vi "Broadcast Single Message.vi"(8 "error in (no error)":errorcluster, 10 "Message In":refnum<class "Message.lvclass">, 11 "Messenger in":refnum<class "Tree-ArrayLocation Queue Messenger.lvclass">) -> (0 "error out":errorcluster, 3 "Messenger out":refnum<class "Tree-ArrayLocation Queue Messenger.lvclass">)   [LabVIEW 2019, in "Tree-ArrayLocation Queue Messenger.lvclass"]
uses:
  Tree-ArrayLocation Queue Messenger.lvclass
  C:/Users/iio/Desktop/NTHU Brain Center/General Purpose/Classes/Ancestor/Messenger/Messenger Composite/Messenger Composite.lvclass
  Ancestor Class/Message/Message.lvclass
  Tree-ArrayLocation Queue Messenger.lvclass/Tree-ArrayLocation Queue Messenger.ctl
  Ancestor Class/Messenger/Messenger Composite/Messenger Composite.lvclass/Messenger Composite.ctl
  Ancestor Class/Messenger/Messenger Composite/Public Data/Read Nodes.vi
  Ancestor Class/Messenger/Messenger/Messenger.lvclass
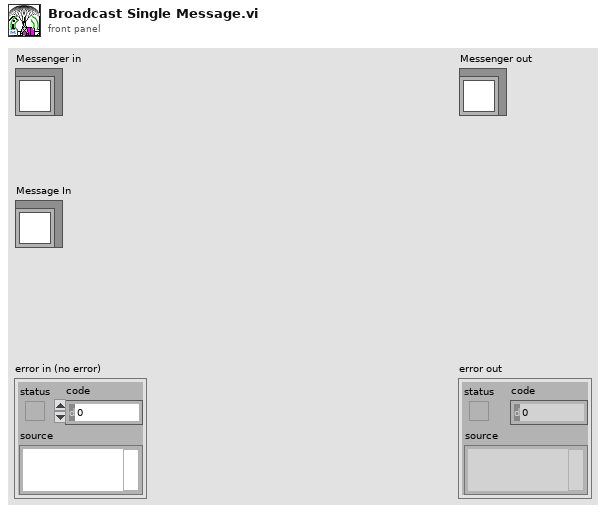
[diagram p1: front panel]
types:
  T1 = typedef "Message Queue.ctl" = refnum<queue>
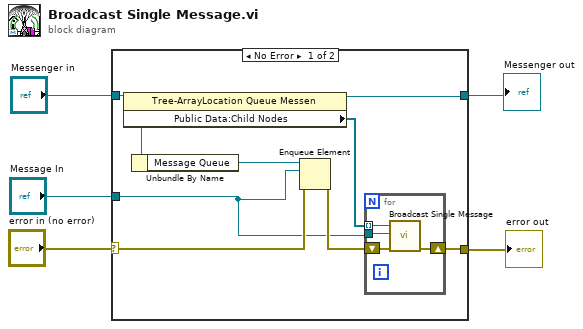
[diagram p0: block diagram]
diagram:
  n1 = case shown="No Error" "error in (no error)" {
    selector: "error in (no error)" -> [w12 w19]
    tunnel: [w10 w19] -> w1
    tunnel: [w7 w18] -> w2
    tunnel: "Messenger in" -> [w8 w18]
    tunnel: "Message In" -> [w9 _]
    frame No Error {
      n2 = property class="Tree-ArrayLocation Queue Messen"(reference=w8) -> (reference out=w7:refnum<class "Tree-ArrayLocation Queue Messenger.lvclass">, "Public Data:Child Nodes"=w6:refnum<class "Messenger.lvclass">[])  [unwired: 1 in, 1 out]
      n3 = Unbundle By Name(w8) -> ("Message Queue"=w13:T1)
      n4 = Enqueue Element(queue=w13, element=w9, error in (no error)=w12) -> (error out=w11:errorcluster)  [unwired: 1 in, 2 out]
      n5 = for {
        shift-right: [w14] -> w10
        shift-left: w11 -> [w15]
        tunnel: w6 -> [w17] mode=indexing
        tunnel: w9 -> [w16]
        n6 = call-dynamic "Broadcast Single Message.vi"("error in (no error)"=w15, "Message In"=w16, "Messenger in"=w17) -> ("error out"=w14:errorcluster)  [unwired: 7 in, 1 out]
      }
    }
    frame Error {
    }
  }
  "error out" <- w1
  "Messenger out" <- w2
